vi "PH_Switch_USB.contents.vi"   [LabVIEW 2014, in "PH_Switch_USB.lvlib"]
doc: "This class is forseen to control easy switches with up to two end position sensors using a NI USB-6008 or 6009 device..\n\nThis class is part of the PHELIX device layer."
uses:
  PH_Switch_USB.lvlib
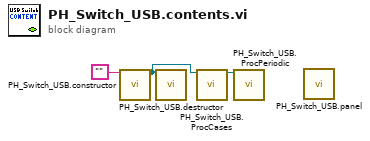
[diagram p0: block diagram]
diagram:
  n1 = call "PH_Switch_USB.constructor.vi"("name"="") -> ("i ref out"=w1:refnum<vi>)  [unwired: 16 in, 2 out]
  n2 = call "PH_Switch_USB.destructor.vi"("i ref in"=w1) -> ()  [unwired: 18 in, 1 out]
  n3 = call "PH_Switch_USB.ProcCases.vi"("i ref in"=w1) -> ("i ref out"=w3:refnum<vi>)  [unwired: 16 in, 2 out]
  n4 = call "PH_Switch_USB.ProcPeriodic.vi"("i ref in"=w3) -> ()  [unwired: 16 in, 3 out]
  n5 = call "PH_Switch_USB.panel.vi"() -> ()  [unwired: 19 in, 1 out]
